vi "_PC_SaveFile window_graph.vi"(6 "signalDataAttr":T1, 8 "error in (no error)":errorcluster, 10 "plot name":string[](array[string]), 11 "XY Graph":cluster{dbl[], sgl[]}[](graph)) -> (0 "error out":errorcluster)   [LabVIEW 2018]
uses:
  PublicSubVI/Class/QMH/QMH.lvclass
  <vilib>/event_ctls.llb/eventvkey.ctl
  <vilib>/Utility/miscctls.llb/LVPoint32TypeDef.ctl
  WindowGraph/window_graph/wfm_feature.lvclass
  WindowGraph/mouse_ctrl/mouse_ctrl.lvclass
  WindowGraph/subVI/mouse_state.ctl
  <vilib>/Utility/miscctls.llb/LVRangeTypeDef.ctl
  PublicSubVI/Class/Sig2MS/ctl/signalDataAttr.ctl
panel:
  in  "shadow graph":cluster{"Array":cluster{"X":dbl, "Y":dbl}[]}[](graph)
  in  "Listbox":i32(listbox)=-1
  in  "Area Plot":string(combo)
  in  "Target plot":string(combo)
  in  "mouse event":T2
  out "Stop":bool
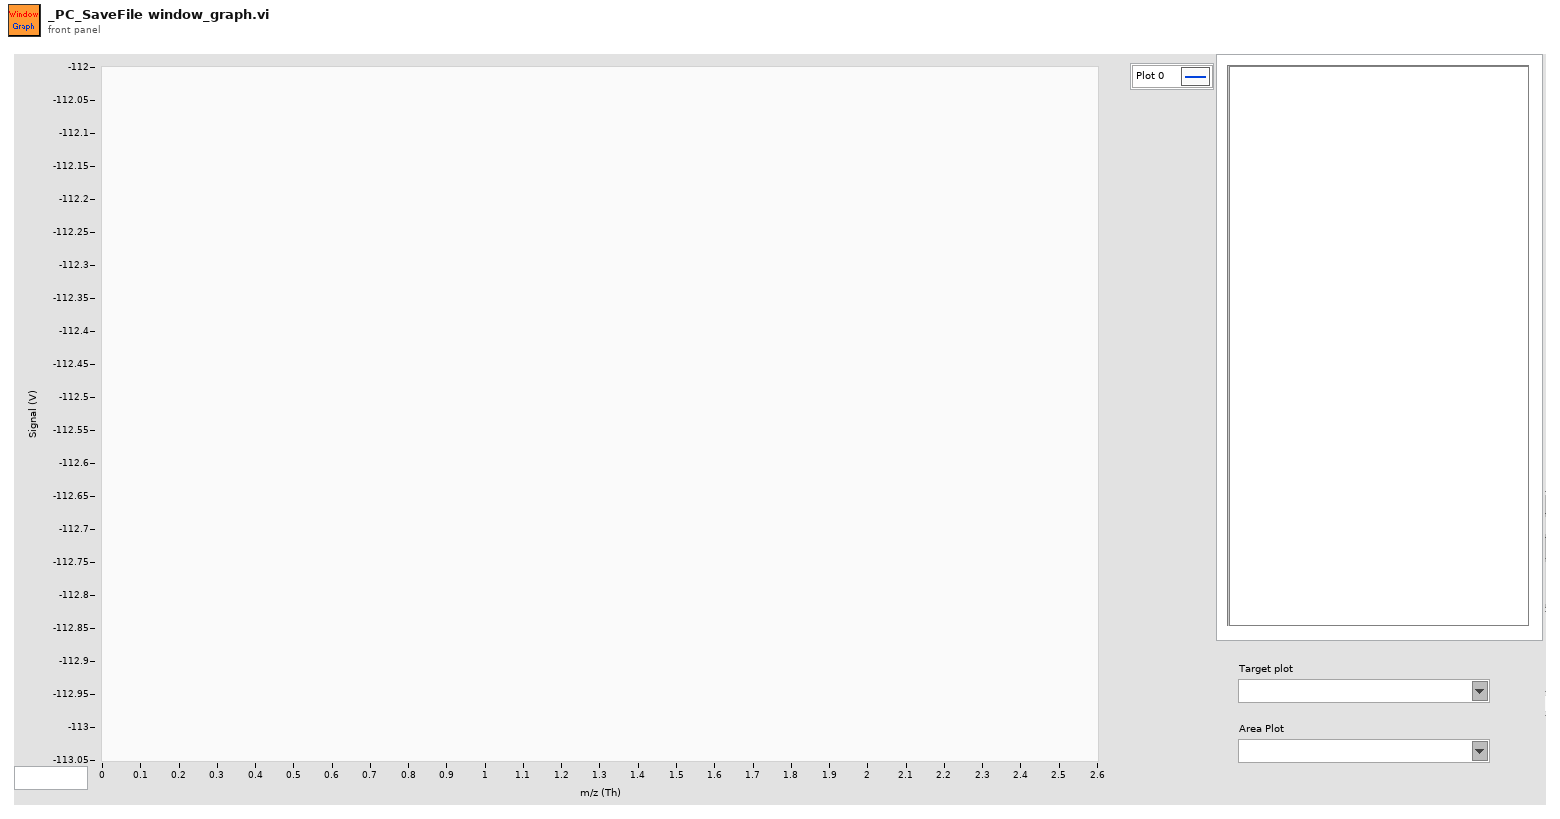
[diagram p1: front panel]
types:
  T1 = typedef "signalDataAttr.ctl" = cluster{"xyXLabel":string, "xyYLabel":string, "wfmXLabel":string, "wfmYLabel":string, "ionXLabel":string, "ionYLabel":string, "dtArr":dbl[]}
  T2 = typedef "mouse_state.ctl" = enum16{"normal", "mouse down", "calc"}
  T3 = cluster{"XY Graph":refnum<vi>, "shadow graph":refnum<vi>, "mouse event":refnum<vi>}
  T4 = typedef "LVRangeTypeDef.ctl" = cluster{"Minimum":dbl, "Maximum":dbl, "Increment":dbl, "Minor Increment":dbl, "Start":dbl}
  T5 = typedef "LVPoint32TypeDef.ctl" = cluster{"Horizontal":i32, "Vertical":i32}
  T6 = cluster{"mouse down pos":cluster{"X":dbl, "Y":dbl}, "mouse up pos":cluster{"X":dbl, "Y":dbl}}
  T7 = cluster{"area":dbl, "height":dbl, "half-height width":dbl}
  T8 = cluster{"baseline data":cluster{"X":dbl, "Y":dbl}[], "vaild region data":cluster{"X":dbl, "Y":dbl}[]}
  T9 = typedef "eventvkey.ctl" = enum16{"ASCII", "Enter", "Return", "Shift", "Ctrl", "Alt", "Cmd", "Opt", "Caps", "NumLock", "Clear", "Break", "Up", "Down", "Left", "Right", "Insert", "Delete", "Home", "End", "PageUp", "PageDown", "Escape", "Help", "Pause", "ScrollLock", "F1", "F2", "F3", "F4", "F5", "F6", "F7", "F8", "F9", "F10", "F11", "F12", "F13", "F14", "F15", "F16", "F17", "F18", "F19", "F20", "F21", "F22", "F23", "F24", "Play", "VolumeUp", "VolumeDown", "Mute", "Two Byte Char"}
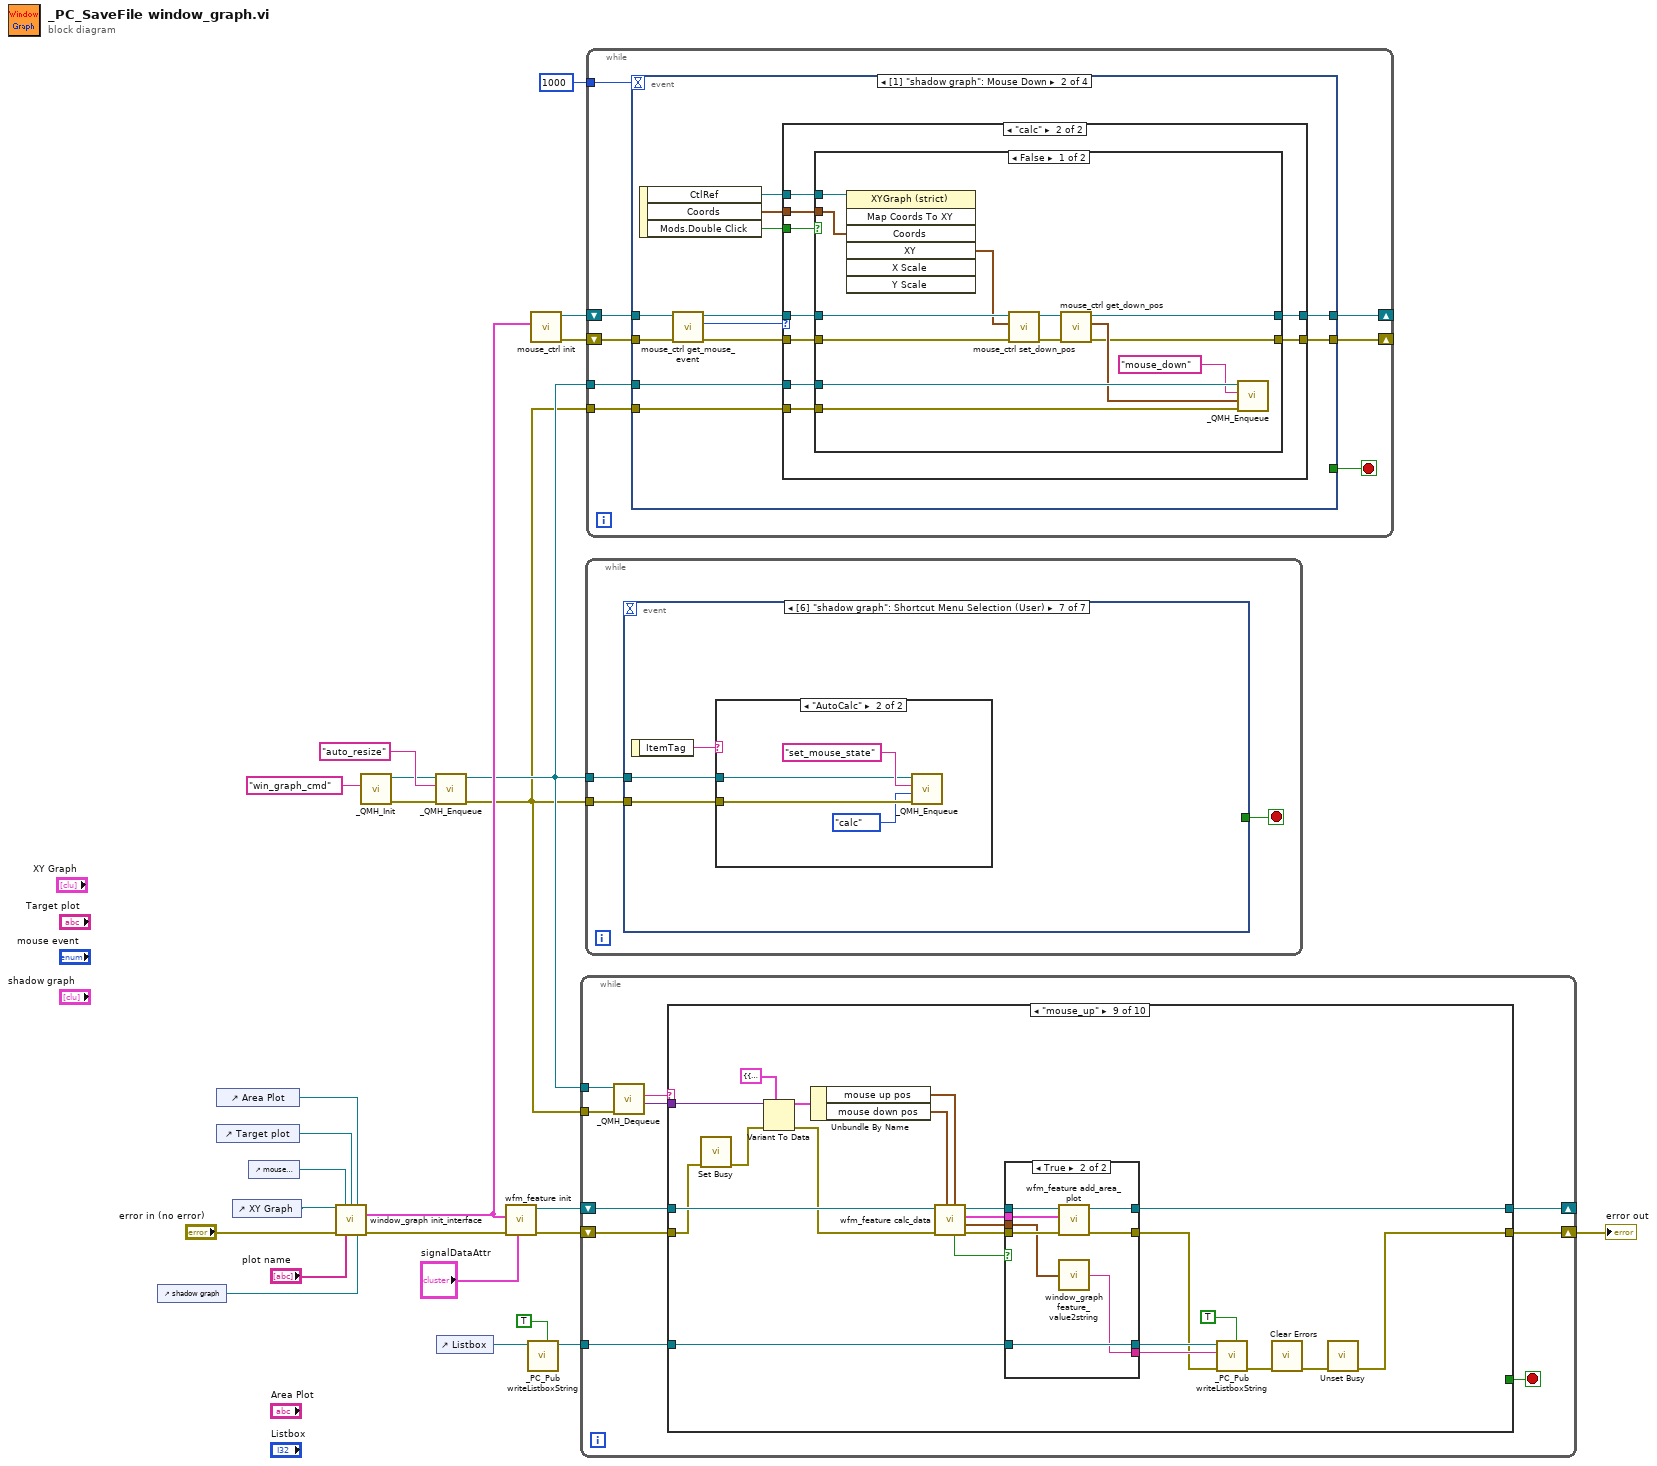
[diagram p0: block diagram]
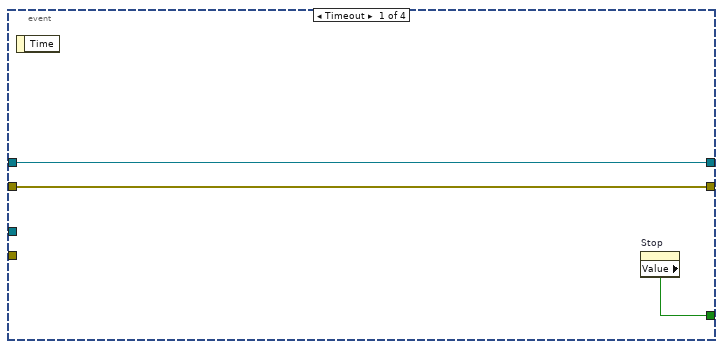
[diagram p2: hidden frame]
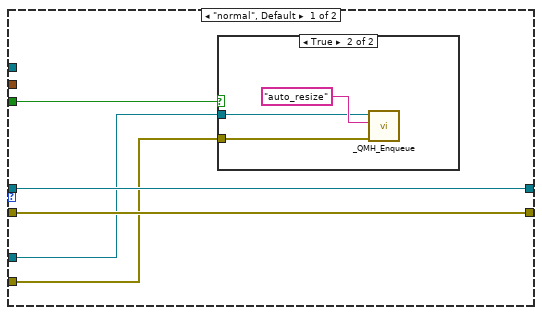
[diagram p3: hidden frame]
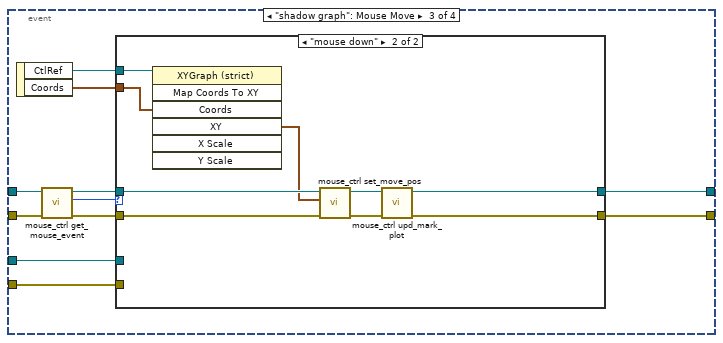
[diagram p6: hidden frame]
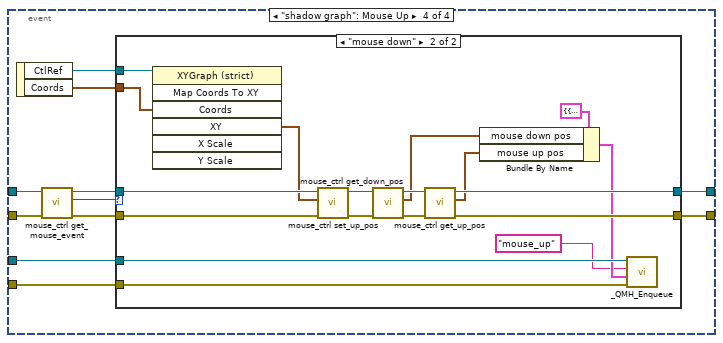
[diagram p8: hidden frame]
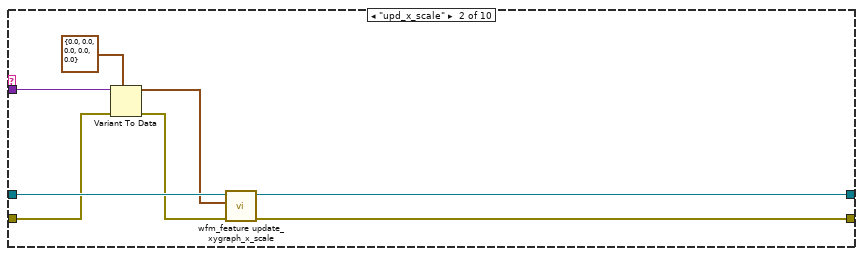
[diagram p11: hidden frame]
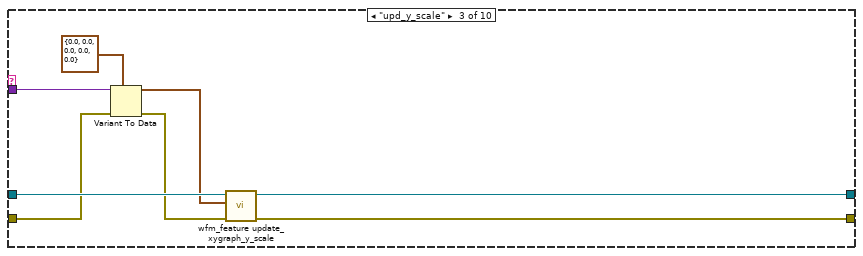
[diagram p12: hidden frame]
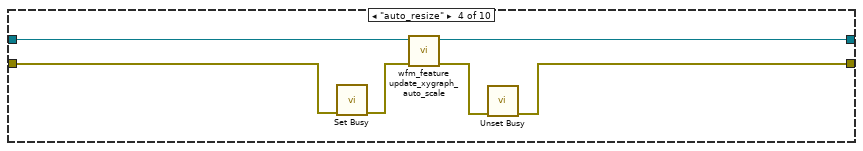
[diagram p13: hidden frame]
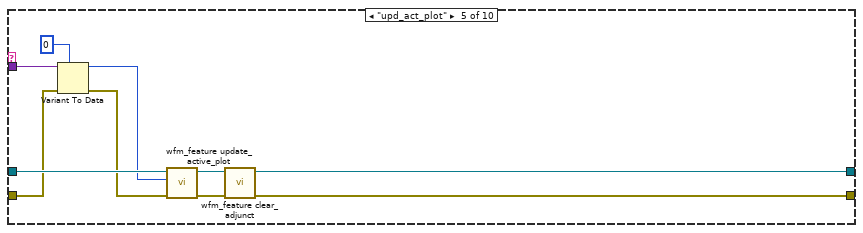
[diagram p14: hidden frame]
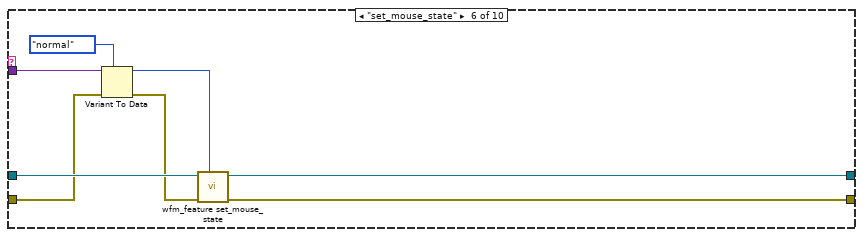
[diagram p15: hidden frame]
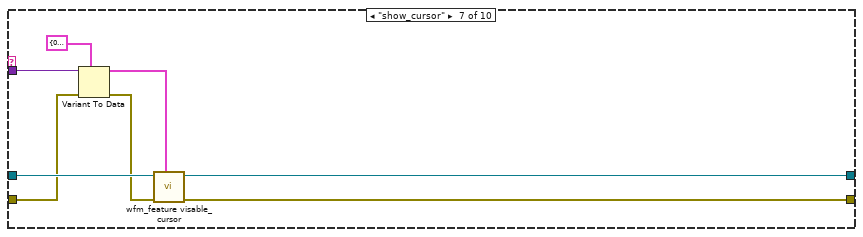
[diagram p16: hidden frame]
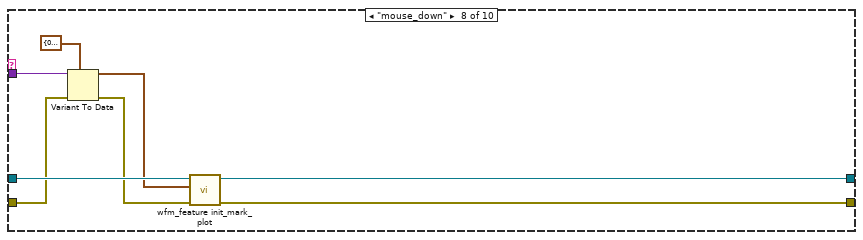
[diagram p17: hidden frame]
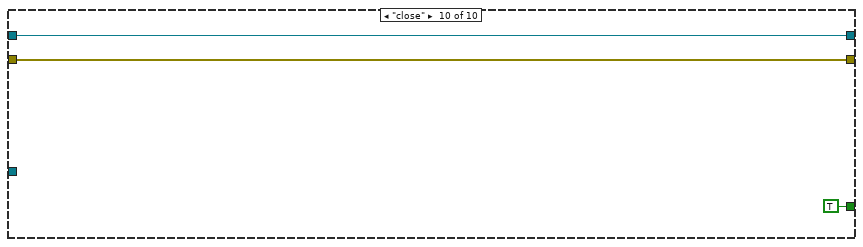
[diagram p19: hidden frame]
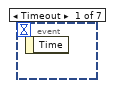
[diagram p20: hidden frame]
diagram:
  n1 = control-ref of="shadow graph"() -> (w4:refnum<vi>)
  n2 = control-ref of="Area Plot"() -> (w2:refnum<vi>)
  n3 = control-ref of="Target plot"() -> (w3:refnum<vi>)
  n4 = control-ref of="XY Graph"() -> (w18:refnum<vi>)
  n5 = control-ref of="mouse event"() -> (w13:refnum<vi>)
  n6 = call "window_graph init_interface.vi"("XY Graph in"=w18, "mouse event"=w13, "Target plot"=w3, "Area Plot"=w2, "error in (no error)"="error in (no error)", "plot name"="plot name", "shadow graph"=w4) -> ("refnum cluster output"=w15:T3, "error out"=w16:errorcluster)  [unwired: 7 in]
  n7 = call "_QMH_Init.vi"("name (unnamed)"="win_graph_cmd") -> ("error out"=w7:errorcluster, "QMH out"=w8:refnum<class "QMH.lvclass">)  [unwired: 9 in]
  n8 = call "_QMH_Enqueue.vi"("error in (no error)"=w7, "Msg"="auto_resize", "QMH in"=w8) -> ("error out"=w5:errorcluster, "QMH out"=w6:refnum<class "QMH.lvclass">)  [unwired: 7 in]
  n9 = control-ref of="Listbox"() -> (w11:refnum<vi>)
  n10 = call "wfm_feature init.vi"("signalDataAttr"="signalDataAttr", "error in (no error)"=w16, "refnum cluster input"=w15) -> ("error out"=w23:errorcluster, "wfm_feature out"=w24:refnum<class "wfm_feature.lvclass">)  [unwired: 7 in]
  n11 = call "_PC_Pub writeListboxString.vi"("Reset (F)"=TRUE, "Listbox Ref Input"=w11) -> ("Listbox Ref Output"=w10:refnum<vi>)  [unwired: 8 in, 1 out]
  n12 = call "mouse_ctrl init.vi"("refnum cluster input"=w15) -> ("error out"=w21:errorcluster, "mouse_ctrl out"=w22:refnum<class "mouse_ctrl.lvclass">)  [unwired: 9 in]
  n13 = while {
    tunnel: w6 -> [w34]
    tunnel: w5 -> [w33]
    shift-right: [w29] -> _
    shift-left: w24 -> [w31]
    shift-right: [w28] -> w14
    shift-left: w23 -> [w30]
    tunnel: w10 -> [w26]
    stop <- w27 stop-if-true
    n14 = call "_QMH_Dequeue.vi"("error in (no error)"=w33, "QMH in"=w34) -> ("Data"=w32:variant, "Msg"=w35:string)  [unwired: 4 in, 4 out]
    n15 = case shown="\"mouse_up\"" w35 {
      tunnel: w32 -> [_ w45 w53 _ w68 w77 w85 w92 w116 _]
      tunnel: w31 -> [w37 w43 w51 w59 w69 w76 w83 w93 w114 w130]
      tunnel: w30 -> [w36 w41 w49 w57 w65 w74 w79 w90 w104 w129]
      tunnel: [w37 w39 w47 w58 w61 w72 w81 w88 w108 w130] -> w29
      tunnel: [w36 w38 w46 w54 w60 w71 w80 w87 w101 w129] -> w28
      tunnel: [_ _ _ _ _ _ _ _ _ TRUE] -> w27
      tunnel: w26 -> [_ _ _ _ _ _ _ _ w100 _]
      frame Default {
      }
      frame "upd_x_scale" {
        n16 = Variant To Data(error in=w41, type=T4 {"Minimum"=0.0, "Maximum"=0.0, "Increment"=0.0, "Minor Increment"=0.0, "Start"=0.0} ("NewRange"), Variant=w45) -> (data=w42:T4, error out=w40:errorcluster)
        n17 = call "wfm_feature update_xygraph_x_scale.vi"("error in (no error)"=w40, "Range"=w42, "wfm_feature in"=w43) -> ("error out"=w38:errorcluster, "wfm_feature out"=w39:refnum<class "wfm_feature.lvclass">)  [unwired: 7 in]
      }
      frame "upd_y_scale" {
        n18 = Variant To Data(error in=w49, type=T4 {"Minimum"=0.0, "Maximum"=0.0, "Increment"=0.0, "Minor Increment"=0.0, "Start"=0.0} ("NewRange"), Variant=w53) -> (data=w50:T4, error out=w48:errorcluster)
        n19 = call "wfm_feature update_xygraph_y_scale.vi"("error in (no error)"=w48, "NewRange"=w50, "wfm_feature in"=w51) -> ("error out"=w46:errorcluster, "wfm_feature out"=w47:refnum<class "wfm_feature.lvclass">)  [unwired: 7 in]
      }
      frame "auto_resize" {
        n20 = call <vilib>:"Set Busy.vi"("error in (no error)"=w57) -> ("error out"=w56:errorcluster)  [unwired: 9 in, 1 out]
        n21 = call "wfm_feature update_xygraph_auto_scale.vi"("error in (no error)"=w56, "wfm_feature in"=w59) -> ("error out"=w55:errorcluster, "wfm_feature out"=w58:refnum<class "wfm_feature.lvclass">)  [unwired: 8 in]
        n22 = call <vilib>:"Unset Busy.vi"("error in (no error)"=w55) -> ("error out"=w54:errorcluster)  [unwired: 10 in]
      }
      frame "upd_act_plot" {
        n23 = Variant To Data(error in=w65, type=0 ("index of element"), Variant=w68) -> (data=w66:i32, error out=w64:errorcluster)
        n24 = call "wfm_feature update_active_plot.vi"("error in (no error)"=w64, "index of element"=w66, "wfm_feature in"=w69) -> ("error out"=w62:errorcluster, "wfm_feature out"=w63:refnum<class "wfm_feature.lvclass">)  [unwired: 7 in]
        n25 = call "wfm_feature clear_adjunct.vi"("error in (no error)"=w62, "wfm_feature in"=w63) -> ("error out"=w60:errorcluster, "wfm_feature out"=w61:refnum<class "wfm_feature.lvclass">)  [unwired: 8 in]
      }
      frame "set_mouse_state" {
        n26 = Variant To Data(error in=w74, type=mouse_state."normal" ("mouse event"), Variant=w77) -> (data=w75:T2, error out=w73:errorcluster)
        n27 = call "wfm_feature set_mouse_state.vi"("mouse event"=w75, "error in (no error)"=w73, "WindowGraph in"=w76) -> ("error out"=w71:errorcluster, "WindowGraph out"=w72:refnum<class "wfm_feature.lvclass">)  [unwired: 7 in]
      }
      frame "show_cursor" {
        n28 = Variant To Data(error in=w79, type=cluster{"Target":i32, "Coords":T5} {"Target"=0, "Coords"={"Horizontal"=0, "Vertical"=0}}, Variant=w85) -> (data=w82:cluster{"Target":i32, "Coords":T5}, error out=w78:errorcluster)
        n29 = call "wfm_feature visable_cursor.vi"("parameter"=w82, "error in (no error)"=w78, "WindowGraph in"=w83) -> ("error out"=w80:errorcluster, "WindowGraph out"=w81:refnum<class "wfm_feature.lvclass">)  [unwired: 7 in]
      }
      frame "mouse_down" {
        n30 = Variant To Data(error in=w90, type=cluster{"X":dbl, "Y":dbl} {"X"=0.0, "Y"=0.0} ("mouse down pos"), Variant=w92) -> (data=w89:cluster{"X":dbl, "Y":dbl}, error out=w86:errorcluster)
        n31 = call "wfm_feature init_mark_plot.vi"("error in (no error)"=w86, "mouse down pos"=w89, "wfm_feature in"=w93) -> ("error out"=w87:errorcluster, "wfm_feature out"=w88:refnum<class "wfm_feature.lvclass">)  [unwired: 7 in]
      }
      frame "mouse_up" {
        n32 = call <vilib>:"Set Busy.vi"("error in (no error)"=w104) -> ("error out"=w103:errorcluster)  [unwired: 9 in, 1 out]
        n33 = Variant To Data(error in=w103, type=T6 {"mouse down pos"={"X"=0.0, "Y"=0.0}, "mouse up pos"={"X"=0.0, "Y"=0.0}}, Variant=w116) -> (data=w112:T6, error out=w113:errorcluster)
        n34 = Unbundle By Name(w112) -> ("mouse up pos"=w110:cluster{"X":dbl, "Y":dbl}, "mouse down pos"=w111:cluster{"X":dbl, "Y":dbl})
        n35 = call "wfm_feature calc_data.vi"("mouse up pos"=w110, "mouse down pos"=w111, "error in (no error)"=w113, "wfm_feature in"=w114) -> ("error out"=w107:errorcluster, "feature cluster"=w94:T7, "fill graph param"=w105:T8, "wfm_feature out"=w109:refnum<class "wfm_feature.lvclass">, "valid"=w106:bool)  [unwired: 3 in]
        n36 = case shown="True" w106 {
          tunnel: w109 -> [w119 w123]
          tunnel: [w119 w127] -> w108
          tunnel: [w118 w126] -> w97
          tunnel: w107 -> [w118 w122]
          tunnel: w105 -> [_ w125]
          tunnel: w100 -> [w117 w124]
          tunnel: [w117 w124] -> w99
          tunnel: [_ w120] -> w98
          tunnel: w94 -> [_ w121]
          frame False {
          }
          frame True {
            n37 = call "wfm_feature add_area_plot.vi"("error in (no error)"=w122, "fill graph param"=w125, "wfm_feature in"=w123) -> ("error out"=w126:errorcluster, "wfm_feature out"=w127:refnum<class "wfm_feature.lvclass">)  [unwired: 7 in]
            n38 = call "window_graph  feature_value2string.vi"("feature cluster"=w121) -> ("feature string"=w120:string)
          }
        }
        n39 = call "_PC_Pub writeListboxString.vi"("Reset (F)"=TRUE, "error in (no error)"=w97, "update_Str"=w98, "Listbox Ref Input"=w99) -> ("error out"=w96:errorcluster)  [unwired: 6 in, 1 out]
        n40 = call <vilib>:"Clear Errors.vi"("error in (no error)"=w96) -> ("error out"=w102:errorcluster)  [unwired: 5 in, 1 out]
        n41 = call <vilib>:"Unset Busy.vi"("error in (no error)"=w102) -> ("error out"=w101:errorcluster)  [unwired: 10 in]
      }
      frame "close" {
      }
    }
  }
  "error out" <- w14
  n42 = while {
    tunnel: w6 -> [w133]
    tunnel: w5 -> [w132]
    stop <- w131 stop-if-true
    n43 = event shown="[6] \"shadow graph\": Shortcut Menu Selection (User)" {
      selector: _ -> [_ _ _ _ _ _ _]
      dyn-events: _ -> [_ _ _ _ _ _ _]
      timeout: _ -> [_ _ _ _ _ _ _]
      tunnel: w133 -> [_ w135 w148 w156 w159 _ w168]
      tunnel: w132 -> [_ w134 w147 w155 w158 _ w167]
      tunnel: [_ _ w146 w154 _ _ _] -> w131
      event Timeout {
        n44 = event-data() -> ()  [unwired: 1 in, 1 out]
      }
      event "shadow graph": Scale Range Change {
        n45 = event-data() -> ("Kind"=w137:enum16{"X-Scale", "Y-Scale", "Z-Scale"}, "NewRange"=w136:T4)  [unwired: 1 in]
        n46 = case shown="\"X-Scale\", Default" w137 {
          tunnel: w136 -> [w139 w143]
          tunnel: w135 -> [w141 w145]
          tunnel: w134 -> [w140 w144]
          frame "Y-Scale" {
            n47 = call "_QMH_Enqueue.vi"("error in (no error)"=w140, "Data"=w139, "Msg"="upd_y_scale", "QMH in"=w141) -> ()  [unwired: 6 in, 2 out]
          }
          frame "X-Scale", Default {
            n48 = call "_QMH_Enqueue.vi"("error in (no error)"=w144, "Data"=w143, "Msg"="upd_x_scale", "QMH in"=w145) -> ()  [unwired: 6 in, 2 out]
          }
        }
      }
      event Key Down? {
        n49 = event-data() -> ("VKey"=w150:T9)  [unwired: 1 in]
        n50 = Equal?(x=w150, y=eventvkey."Escape") -> (x = y?=w146:bool)
        n51 = case shown="True" w146 {
          tunnel: w148 -> [_ w153]
          tunnel: w147 -> [_ w152]
          frame False {
          }
          frame True {
            n52 = call "_QMH_Enqueue.vi"("error in (no error)"=w152, "Msg"="close", "QMH in"=w153) -> ()  [unwired: 7 in, 2 out]
          }
        }
        n53 = event-data("Discard?"=w146) -> ()  [unwired: 1 in, 1 out]
      }
      event Panel Close {
        w154 = TRUE
        n54 = event-data() -> ()  [unwired: 1 in, 1 out]
        n55 = call "_QMH_Enqueue.vi"("error in (no error)"=w155, "Msg"="close", "QMH in"=w156) -> ()  [unwired: 7 in, 2 out]
        "Stop" <- w154
      }
      event "Target plot": Value Change {
        n56 = event-data() -> ("CtlRef"=w166:refnum<vi>, "NewVal"=w164:string)  [unwired: 1 in]
        n57 = property class="CmbBox"(reference=w166) -> ("Strings[]"=w165:string[])  [unwired: 1 in, 2 out]
        n58 = Equal?(x=w165, y=w164) -> (x = y?=w163:bool[])
        n59 = Search 1D Array(1D array=w163, element=TRUE) -> (index of element=w160:i32)  [unwired: 1 in]
        n60 = call "_QMH_Enqueue.vi"("error in (no error)"=w158, "Data"=w160, "Msg"="upd_act_plot", "QMH in"=w159) -> ()  [unwired: 6 in, 2 out]
      }
      event "Area Plot": Value Change {
        n61 = event-data() -> ()  [unwired: 1 in, 2 out]
      }
      event "shadow graph": Shortcut Menu Selection (User) {
        n62 = event-data() -> ("ItemTag"=w169:string)  [unwired: 1 in]
        n63 = case shown="\"AutoCalc\"" w169 {
          tunnel: w168 -> [_ w172]
          tunnel: w167 -> [_ w171]
          frame "False", Default {
          }
          frame "AutoCalc" {
            n64 = call "_QMH_Enqueue.vi"("error in (no error)"=w171, "Data"=mouse_state."calc" ("mouse event"), "Msg"="set_mouse_state", "QMH in"=w172) -> ()  [unwired: 6 in, 2 out]
          }
        }
      }
    }
  }
  n65 = while {
    tunnel: 1000 -> [w179]
    tunnel: w6 -> [w177]
    tunnel: w5 -> [w176]
    shift-right: [w175] -> _
    shift-left: w22 -> [w181]
    shift-right: [w174] -> _
    shift-left: w21 -> [w180]
    stop <- w178 stop-if-true
    n66 = event shown="[1] \"shadow graph\": Mouse Down" {
      selector: _ -> [_ _ _ _]
      dyn-events: _ -> [_ _ _ _]
      timeout: w179 -> [_ _ _ _]
      tunnel: w181 -> [w183 w193 w236 w258]
      tunnel: w180 -> [w182 w192 w235 w257]
      tunnel: [w184 _ _ _] -> w178
      tunnel: w177 -> [_ w196 w239 w261]
      tunnel: w176 -> [_ w195 w238 w260]
      tunnel: [w183 w187 w230 w252] -> w175
      tunnel: [w182 w186 w229 w251] -> w174
      event Timeout {
        n67 = event-data() -> ()  [unwired: 1 in, 1 out]
        n68 = property on="Stop" class="Bool (strict)"() -> ("Value"=w184:bool)  [unwired: 2 in, 2 out]
      }
      event "shadow graph": Mouse Down {
        n69 = event-data() -> ("CtlRef"=w188:refnum<vi>, "Coords"=w194:T5, "Mods.Double Click"=w185:bool)  [unwired: 1 in]
        n70 = call "mouse_ctrl get_mouse_event.vi"("error in (no error)"=w192, "mouse_ctrl in"=w193) -> ("error out"=w189:errorcluster, "mouse event"=w191:T2, "mouse_ctrl out"=w190:refnum<class "mouse_ctrl.lvclass">)  [unwired: 7 in]
        n71 = case shown="\"calc\"" w191 {
          tunnel: w196 -> [w198 w213]
          tunnel: w195 -> [w197 w212]
          tunnel: w194 -> [_ w208]
          tunnel: w190 -> [w201 w211]
          tunnel: w189 -> [w200 w210]
          tunnel: w188 -> [_ w209]
          tunnel: [w201 w207] -> w187
          tunnel: [w200 w206] -> w186
          tunnel: w185 -> [w199 w205]
          frame "normal", Default {
            n72 = case shown="True" w199 {
              tunnel: w198 -> [_ w203]
              tunnel: w197 -> [_ w202]
              frame False {
              }
              frame True {
                n73 = call "_QMH_Enqueue.vi"("error in (no error)"=w202, "Msg"="auto_resize", "QMH in"=w203) -> ()  [unwired: 7 in, 2 out]
              }
            }
          }
          frame "calc" {
            n74 = case shown="False" w205 {
              tunnel: w213 -> [w226 _]
              tunnel: w212 -> [w225 _]
              tunnel: w211 -> [w220 w228]
              tunnel: w210 -> [w219 w227]
              tunnel: w209 -> [w218 _]
              tunnel: w208 -> [w217 _]
              tunnel: [w215 w228] -> w207
              tunnel: [w214 w227] -> w206
              frame False {
                n75 = invoke class="XYGraph (strict)" method="Map Coords To XY"(reference=w218, "Coords"=w217) -> ("XY"=w216:cluster{"X":dbl, "Y":dbl})  [unwired: 5 in, 6 out]
                n76 = call "mouse_ctrl set_down_pos.vi"("error in (no error)"=w219, "xy pos"=w216, "mouse_ctrl in"=w220) -> ("error out"=w222:errorcluster, "mouse_ctrl out"=w223:refnum<class "mouse_ctrl.lvclass">)  [unwired: 7 in]
                n77 = call "mouse_ctrl get_down_pos.vi"("error in (no error)"=w222, "mouse_ctrl in"=w223) -> ("error out"=w214:errorcluster, "mouse down pos"=w221:cluster{"X":dbl, "Y":dbl}, "mouse_ctrl out"=w215:refnum<class "mouse_ctrl.lvclass">)  [unwired: 7 in]
                n78 = call "_QMH_Enqueue.vi"("error in (no error)"=w225, "Data"=w221, "Msg"="mouse_down", "QMH in"=w226) -> ()  [unwired: 6 in, 2 out]
              }
              frame True {
              }
            }
          }
        }
      }
      event "shadow graph": Mouse Move {
        n79 = event-data() -> ("CtlRef"=w231:refnum<vi>, "Coords"=w237:T5)  [unwired: 1 in]
        n80 = call "mouse_ctrl get_mouse_event.vi"("error in (no error)"=w235, "mouse_ctrl in"=w236) -> ("error out"=w232:errorcluster, "mouse event"=w234:T2, "mouse_ctrl out"=w233:refnum<class "mouse_ctrl.lvclass">)  [unwired: 7 in]
        n81 = case shown="\"mouse down\"" w234 {
          tunnel: w239 -> [_ _]
          tunnel: w238 -> [_ _]
          tunnel: w237 -> [_ w249]
          tunnel: w233 -> [w241 w247]
          tunnel: w232 -> [w240 w245]
          tunnel: w231 -> [_ w250]
          tunnel: [w241 w243] -> w230
          tunnel: [w240 w242] -> w229
          frame "normal", Default {
          }
          frame "mouse down" {
            n82 = invoke class="XYGraph (strict)" method="Map Coords To XY"(reference=w250, "Coords"=w249) -> ("XY"=w246:cluster{"X":dbl, "Y":dbl})  [unwired: 5 in, 6 out]
            n83 = call "mouse_ctrl set_move_pos.vi"("error in (no error)"=w245, "xy pos"=w246, "mouse_ctrl in"=w247) -> ("error out"=w248:errorcluster, "mouse_ctrl out"=w244:refnum<class "mouse_ctrl.lvclass">)  [unwired: 7 in]
            n84 = call "mouse_ctrl upd_mark_plot.vi"("error in (no error)"=w248, "mouse_ctrl in"=w244) -> ("error out"=w242:errorcluster, "mouse_ctrl out"=w243:refnum<class "mouse_ctrl.lvclass">)  [unwired: 8 in]
          }
        }
      }
      event "shadow graph": Mouse Up {
        n85 = event-data() -> ("CtlRef"=w253:refnum<vi>, "Coords"=w259:T5)  [unwired: 1 in]
        n86 = call "mouse_ctrl get_mouse_event.vi"("error in (no error)"=w257, "mouse_ctrl in"=w258) -> ("error out"=w254:errorcluster, "mouse event"=w256:T2, "mouse_ctrl out"=w255:refnum<class "mouse_ctrl.lvclass">)  [unwired: 7 in]
        n87 = case shown="\"mouse down\"" w256 {
          tunnel: w261 -> [_ w267]
          tunnel: w260 -> [_ w266]
          tunnel: w259 -> [_ w280]
          tunnel: w255 -> [w263 w279]
          tunnel: w254 -> [w262 w277]
          tunnel: w253 -> [_ w281]
          tunnel: [w263 w272] -> w252
          tunnel: [w262 w271] -> w251
          frame "normal", Default {
          }
          frame "mouse down" {
            n88 = invoke class="XYGraph (strict)" method="Map Coords To XY"(reference=w281, "Coords"=w280) -> ("XY"=w278:cluster{"X":dbl, "Y":dbl})  [unwired: 5 in, 6 out]
            n89 = call "mouse_ctrl set_up_pos.vi"("error in (no error)"=w277, "xy pos"=w278, "mouse_ctrl in"=w279) -> ("error out"=w275:errorcluster, "mouse_ctrl out"=w276:refnum<class "mouse_ctrl.lvclass">)  [unwired: 7 in]
            n90 = call "mouse_ctrl get_down_pos.vi"("error in (no error)"=w275, "mouse_ctrl in"=w276) -> ("error out"=w273:errorcluster, "mouse down pos"=w268:cluster{"X":dbl, "Y":dbl}, "mouse_ctrl out"=w274:refnum<class "mouse_ctrl.lvclass">)  [unwired: 7 in]
            n91 = call "mouse_ctrl get_up_pos.vi"("error in (no error)"=w273, "mouse_ctrl in"=w274) -> ("error out"=w271:errorcluster, "mouse up pos"=w269:cluster{"X":dbl, "Y":dbl}, "mouse_ctrl out"=w272:refnum<class "mouse_ctrl.lvclass">)  [unwired: 7 in]
            n92 = Bundle By Name(cluster=T6 {"mouse down pos"={"X"=0.0, "Y"=0.0}, "mouse up pos"={"X"=0.0, "Y"=0.0}}, "mouse down pos"=w268, "mouse up pos"=w269) -> (w265:T6)
            n93 = call "_QMH_Enqueue.vi"("error in (no error)"=w266, "Data"=w265, "Msg"="mouse_up", "QMH in"=w267) -> ()  [unwired: 6 in, 2 out]
          }
        }
      }
    }
  }
